vi "Make Prediction.vi"(0 "Model_Predictor in":refnum<class "Model_Predictor.lvclass">, 5 "Assumend_control":bool, 9 "Last PWM On":i32, 11 "error in (no error)":errorcluster) -> (4 "Model_Predictor out":refnum<class "Model_Predictor.lvclass">, 6 "Achieved min or max":dbl, 8 "Controls":i16[](array[numeric]), 10 "Array":dbl[](array[numeric]), 15 "error out":errorcluster)   [LabVIEW 2021, in "MBPOnOff_Controller.lvlib" / "Model_Predictor.lvclass"]
uses:
  Model_Predictor.lvclass
  Model_Predictor.lvclass/Model_Predictor.ctl
panel:
  out "Numeric":i32
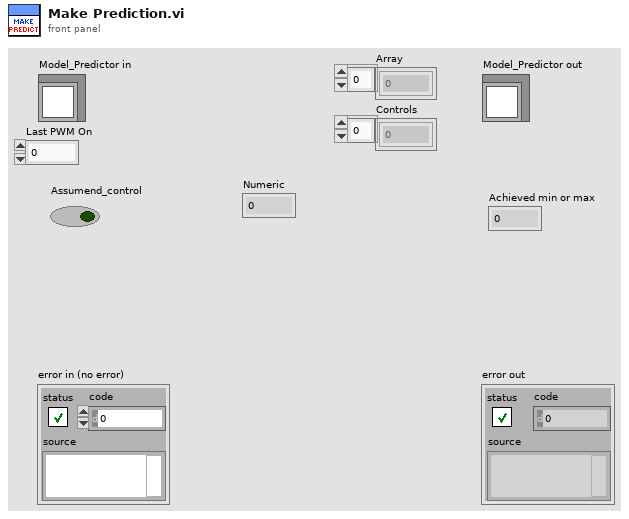
[diagram p1: front panel]
types:
  T1 = typedef "MBPOnOff_Controller.lvlib/Model_Predictor.lvclass/state_variables.ctl" = cluster{"So":dbl, "kLa":dbl}
  T2 = typedef "MBPOnOff_Controller.lvlib/Model_Predictor.lvclass/Model_v1_parameters.ctl" = cluster{"Sosat":dbl, "OUR":dbl, "R_OUR":dbl, "T_kLa":dbl, "R_T_kLa":dbl, "T0":dbl, "ku":dbl, "dt":dbl, "PWM total period":dbl, "PWM ON period":dbl, "OUR calc period":dbl, "OUR calc threshold":dbl}
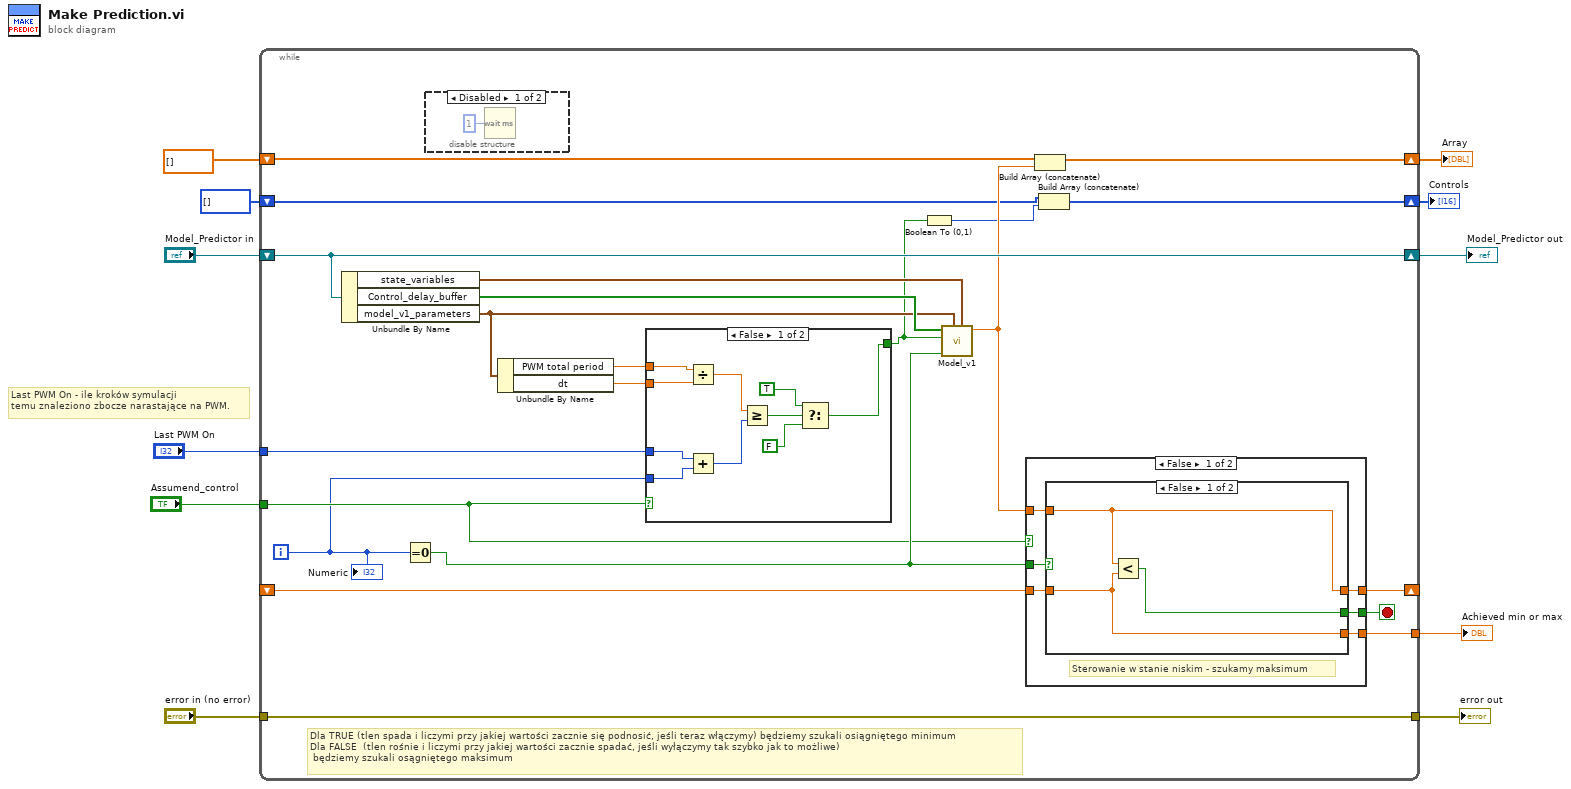
[diagram p0: block diagram]
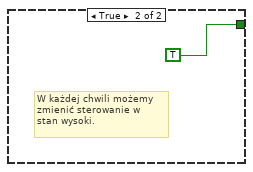
[diagram p2: hidden frame]
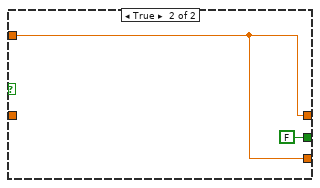
[diagram p4: hidden frame]
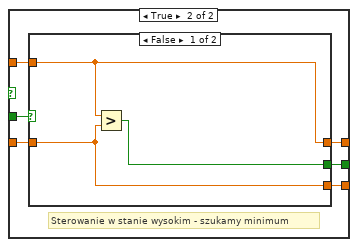
[diagram p5: hidden frame]
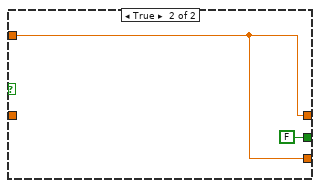
[diagram p6: hidden frame]
diagram:
  # "Last PWM On - ile kroków symulacji\ntemu znaleziono zbocze narastające na PWM."
  n1 = while {
    shift-right: [w32] -> w10
    shift-left: "Model_Predictor in" -> [w32]
    tunnel: "error in (no error)" -> [w33]
    tunnel: [w33] -> w8
    tunnel: "Assumend_control" -> [w20]
    shift-right: [w29] -> _
    shift-left: _ -> [w28]
    tunnel: [w27] -> w6
    shift-right: [w25] -> w4
    shift-left: dbl[] [] -> [w26]
    tunnel: "Last PWM On" -> [w17]
    shift-right: [w13] -> w1
    shift-left: i16[] [] -> [w12]
    i -> [w16]
    stop <- w30 stop-if-true
    # "Dla TRUE (tlen spada i liczymi przy jakiej wartości zacznie się podnosić, jeśli teraz włączymy) będziemy szukali osiągniętego minimum\nDla FALSE  (tlen rośnie i liczymi przy jakiej wartości zacznie spadać, jeśli wyłączymy tak szybko jak to możliwe)\n będziemy szukali osągniętego maksimum"
    n2 = Unbundle By Name(w32) -> ("state_variables"=w23:T1, "Control_delay_buffer"=w22:bool[], "model_v1_parameters"=w21:T2)
    n3 = Equal To 0?(x=w16) -> (x = 0?=w31:bool)
    n4 = disable-structure shown="Disabled" {
      frame Disabled {
        n5 = Wait (ms)(milliseconds to wait=u32 1) -> ()  [unwired: 1 out]
      }
      frame Enabled {
      }
    }
    n6 = Unbundle By Name(w21) -> ("PWM total period"=w19:dbl, "dt"=w18:dbl)
    n7 = case shown="False" w20 {
      tunnel: w19 -> [w41 _]
      tunnel: w18 -> [w40 _]
      tunnel: w17 -> [w43 _]
      tunnel: w16 -> [w42 _]
      tunnel: [w34 TRUE] -> w15
      frame False {
        n8 = Divide(x=w41, y=w40) -> (x/y=w39:dbl)
        n9 = Add(x=w43, y=w42) -> (x+y=w38:i32)
        n10 = Greater Or Equal?(x=w39, y=w38) -> (x >= y?=w37:bool)
        n11 = Select(t=TRUE, s=w37, f=FALSE) -> (s? t:f=w34:bool)
      }
      frame True {
        # "W każdej chwili możemy\nzmienić sterowanie w\nstan wysoki."
      }
    }
    n12 = Boolean To (0,1)(Boolean=w15) -> (0, 1=w14:i16)
    n13 = call "Model_v1.vi"("state_variables"=w23, "model_v1_parameters"=w21, "init?"=w31, "assumed_U"=w15, "Control delay buffer"=w22) -> ("Y_out"=w24:dbl)  [unwired: 6 in]
    n14 = case shown="False" w20 {
      tunnel: w31 -> [w46 w62]
      tunnel: [w49 w61] -> w30
      tunnel: w24 -> [w51 w60]
      tunnel: [w48 w59] -> w29
      tunnel: w28 -> [w50 w58]
      tunnel: [w47 w57] -> w27
      frame False {
        # "Sterowanie w stanie niskim - szukamy maksimum"
        n15 = case shown="False" w46 {
          tunnel: [w52 FALSE] -> w49
          tunnel: w51 -> [w54 w55]
          tunnel: [w54 w55] -> w48
          tunnel: w50 -> [w53 _]
          tunnel: [w53 w55] -> w47
          frame False {
            n16 = Less?(x=w54, y=w53) -> (x < y?=w52:bool)
          }
          frame True {
          }
        }
      }
      frame True {
        # "Sterowanie w stanie wysokim - szukamy minimum"
        n17 = case shown="False" w62 {
          tunnel: [w63 FALSE] -> w61
          tunnel: w60 -> [w65 w66]
          tunnel: [w65 w66] -> w59
          tunnel: w58 -> [w64 _]
          tunnel: [w64 w66] -> w57
          frame False {
            n18 = Greater?(x=w65, y=w64) -> (0:w63:bool)
          }
          frame True {
          }
        }
      }
    }
    n19 = Build Array (concatenate)(w26, w24) -> (w25:dbl[])
    n20 = Build Array (concatenate)(w12, w14) -> (w13:i16[])
    "Numeric" <- w16
  }
  "error out" <- w8
  "Model_Predictor out" <- w10
  "Achieved min or max" <- w6
  "Array" <- w4
  "Controls" <- w1
